vi "Write_DO_Module.vi"(8 "error in (no error)":errorcluster, 10 "DO_Value":u32, 11 "USB-87Pn in":refnum<class "USB-87Pn.lvclass">) -> (0 "error out":errorcluster, 3 "USB-87Pn out":refnum<class "USB-87Pn.lvclass">)   [LabVIEW 2019, in "USB-87Pn.lvlib" / "USB-87Pn.lvclass"]
uses:
  USB-87Pn.lvclass
  USB-87Pn.lvclass/USB-87Pn.ctl
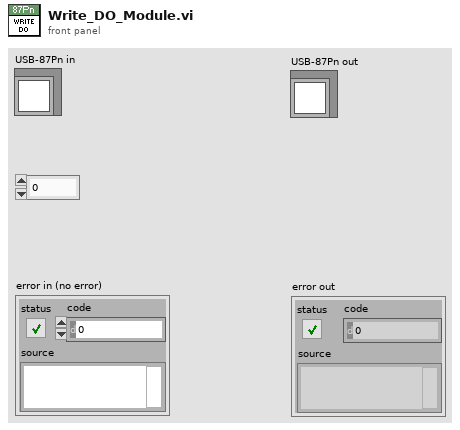
[diagram p1: front panel]
types:
  T1 = typedef "USB-87Pn.lvlib/USB-87Pn.lvclass/DO_Module_Data.ctl" = cluster{"Module_Data":T2, "DO_Channels":cluster{"Enabled":bool, "Alias":string}[]}
  T2 = typedef "USB-87Pn.lvlib/USB-87Pn.lvclass/Module_Data.ctl" = cluster{"Number of Channels":u8, "Address":i16, "Alias":string}
  T3 = cluster{"ComPort":u8, "Address":i16, "Slot":i16, "CheckSum":i16, "TimeOut":i16}
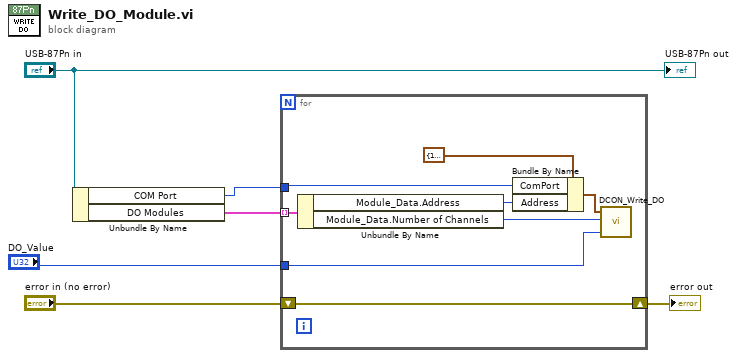
[diagram p0: block diagram]
diagram:
  n1 = Unbundle By Name("USB-87Pn in") -> ("COM Port"=w3:u8, "DO Modules"=w4:T1[])
  n2 = for {
    tunnel: w4 -> [w14] mode=indexing
    tunnel: "DO_Value" -> [w8]
    tunnel: w3 -> [w12]
    shift-right: [w7] -> w2
    shift-left: "error in (no error)" -> [w7]
    n3 = Unbundle By Name(w14) -> ("Module_Data.Address"=w13:i16, "Module_Data.Number of Channels"=w9:u8)
    n4 = Bundle By Name(cluster=T3 {"ComPort"=1, "Address"=0, "Slot"=-1, "CheckSum"=0, "TimeOut"=1000} ("DCON_Module"), "ComPort"=w12, "Address"=w13) -> (w10:T3)
    n5 = call <vilib>:"DCON_Write_DO.vi"("DO_Value"=w8, "DOTotalCh"=w9, "DCON_Module"=w10) -> ()  [unwired: 2 in, 1 out]
  }
  "error out" <- w2
  "USB-87Pn out" <- "USB-87Pn in"
